vi "Calibrate_Plates.vi"() -> ()   [LabVIEW 2013]
uses:
  <vilib>/rvi/interface/nirviOpenFPGA/nirviOpenFPGA.xnode
  <vilib>/rvi/interface/nirviReadWriteControl/nirviReadWriteControl.xnode
  NiFpgaLv.dll
  <vilib>/Utility/error.llb/Error Cluster From Error Code.vi
  <vilib>/rvi/interface/Simulation/niFpgaSimulationCallBeginRW.vi
  <vilib>/rvi/errors/niLvFpgaAdjustHostInterfaceError.vi
  <vilib>/rvi/interface/nirviMethod/nirviMethod.xnode
  <vilib>/FPGAPlugInAG/Dynamic/niLvFpga_Run_Dynamic.vi
  <vilib>/rvi/interface/nirviCloseFPGA/nirviCloseFPGA.xnode
  <vilib>/FPGAPlugInAG/Dynamic/niLvFpga_Close_Dynamic.vi
  FPGA Bitfiles/ProjetoTasca_FPGATarget_ProjetoTASCA_c15+uw0dO0I.lvbitx
  ProjetoTASCA.vi
  <vilib>/rvi/interface/nirviMethod/StockFPGA_InlinedMethodWaitForSingleIRQ.vi
  <vilib>/FPGAPlugInAG/Dynamic/niLvFpga_WaitOnIrq_Dynamic.vi
  <vilib>/FPGAPlugInAG/cRIO-9075/niLvFpga_Open_cRIO-9075.vi
  <vilib>/rvi/interface/common/dynamic/niFpgaDynamicAddResources.vi
panel:
  in  "Passo da placa":dbl=0.5 format="%#_13g"
  out "Posicao da Placa":dbl format="%#_13g"
  in  "Arquivo de Saida":path=path "C:/SteeringDistillation/Medidas"
  out "Contagens - Det. 1":u32
  in  "Measurement Time (s)":sgl=1.0
  in  "Placa a calibrar":u16=1
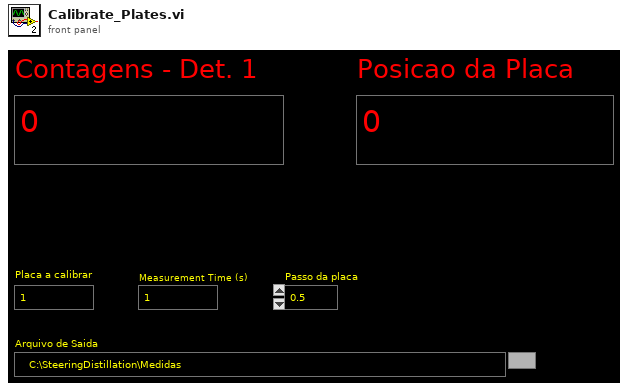
[diagram p1: front panel]
types:
  T1 = enum16{"open", "replace", "create", "open or create", "replace or create", "replace or create with confirmation"}
  T2 = cluster{"connection TCP":refnum<k5>, "LogTo File":bool, "Log File refnum":refnum<file>, "no error if error log":bool}
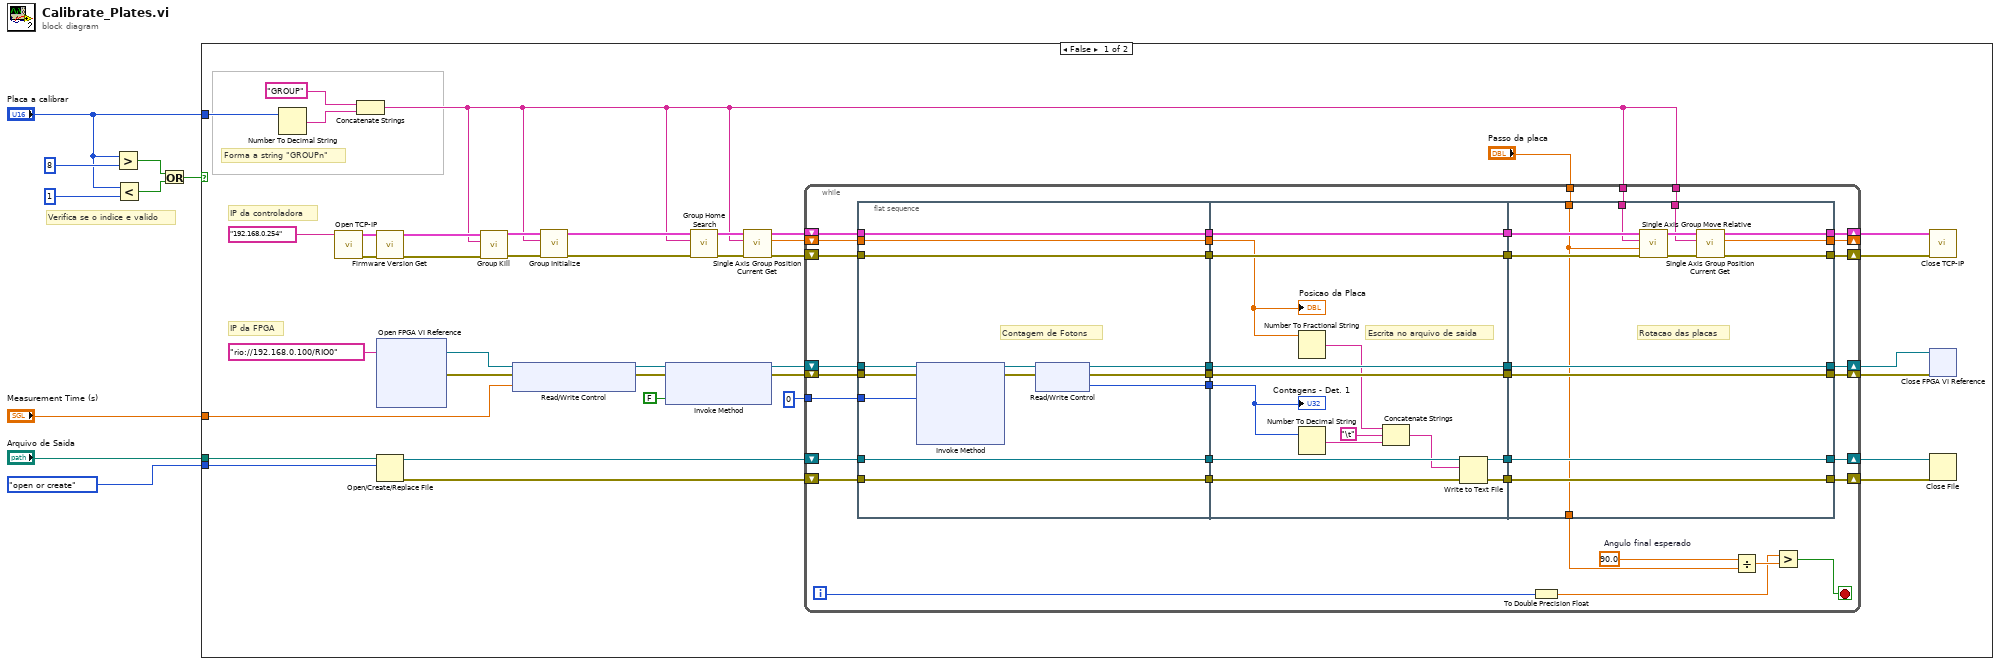
[diagram p0: block diagram]
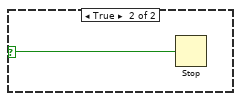
[diagram p2: hidden frame]
diagram:
  # "Verifica se o indice e valido"
  n1 = Greater?(x="Placa a calibrar", y=u16 8) -> (0:w7:bool)
  n2 = Less?(x="Placa a calibrar", y=u16 1) -> (x < y?=w6:bool)
  n3 = Or(x=w7, y=w6) -> (x .or. y?=w5:bool)
  n4 = case shown="False" w5 {
    selector: w5 -> [_ w126]
    tunnel: "Placa a calibrar" -> [w46 _]
    tunnel: "Measurement Time (s)" -> [w31 _]
    tunnel: T1."open or create" -> [w21 _]
    tunnel: "Arquivo de Saida" -> [w20 _]
    frame False {
      # "IP da FPGA"
      # "Forma a string \"GROUPn\""
      # "IP da controladora"
      n5 = Number To Decimal String(number=w46) -> (decimal integer string=w48:string)  [unwired: 1 in]
      n6 = call <userlib>:"Open TCP-IP.vi"("address"="192.168.0.254") -> ("error out"=w44:errorcluster, "Connection ID"=w43:T2)  [unwired: 8 in, 1 out]
      n7 = Concatenate Strings("GROUP" ("Group Name (250 c max)"), w48) -> (w10:string)
      n8 = call <userlib>:"Firmware Version Get.vi"("error in (no error)"=w44, "connection ID in"=w43) -> ("error out"=w41:errorcluster, "connection ID out"=w42:T2)  [unwired: 6 in, 2 out]
      n9 = xnode "Open FPGA VI Reference"("resource name"=tag "rio://192.168.0.100/RIO0") -> ("FPGA VI Reference Out"=w36:refnum<k20>, "error out"=w35:errorcluster)  [unwired: 1 in]
      n10 = Open/Create/Replace File(file path (use dialog)=w20, operation (0:open)=w21) -> (refnum out=w22:refnum<file>, error out=w23:errorcluster)  [unwired: 4 in, 1 out]
      n11 = call <userlib>:"Group Kill.vi"("error in (no error)"=w41, "Group Name (250 c max)"=w10, "connection ID in"=w42) -> ("error out"=w39:errorcluster, "connection ID out"=w40:T2)  [unwired: 6 in, 1 out]
      n12 = xnode "Read/Write Control"("FPGA VI Reference In"=w36, "error in"=w35, "Measurement Time (s)"=w31) -> ("FPGA VI Reference Out"=w34:refnum<k20>, "error out"=w33:errorcluster)
      n13 = call <userlib>:"Group Initialize.vi"("error in (no error)"=w39, "Group Name (250 c max)"=w10, "connection ID in"=w40) -> ("error out"=w11:errorcluster, "connection ID out"=w38:T2)  [unwired: 6 in, 1 out]
      n14 = xnode "Invoke Method"("FPGA VI Reference In"=w34, "error in"=w33, "Wait Until Done (F)"=FALSE) -> ("FPGA VI Reference Out"=w27:refnum<k20>, "error out"=w28:errorcluster)
      n15 = call <userlib>:"Group Home Search.vi"("error in (no error)"=w11, "Group Name (250 c max)"=w10, "connection ID in"=w38) -> ("error out"=w16:errorcluster, "connection ID out"=w17:T2)  [unwired: 6 in, 1 out]
      n16 = call <userlib>:"Single Axis Group Position Current Get.vi"("error in (no error)"=w16, "Group  Name (250 c max)"=w10, "connection ID in"=w17) -> ("error out"=w14:errorcluster, "Current Position (units)"=w13:dbl, "connection ID out"=w15:T2)  [unwired: 5 in, 1 out]
      n17 = while {
        tunnel: w10 -> [w81]
        tunnel: w10 -> [w76]
        tunnel: 0 ("IRQ Number(s)") -> [w86]
        shift-right: [w85] -> w29
        shift-left: w28 -> [w84]
        shift-right: [w82] -> w26
        shift-left: w27 -> [w83]
        shift-right: [w78] -> w25
        shift-left: w22 -> [w80]
        shift-right: [w77] -> w24
        shift-left: w23 -> [w79]
        shift-right: [w73] -> w19
        shift-left: w15 -> [w74]
        shift-right: [w72] -> w18
        shift-left: w14 -> [w75]
        shift-right: [w57] -> _
        shift-left: w13 -> [w71]
        tunnel: "Passo da placa" -> [w56]
        i -> [w50]
        stop <- w51 stop-if-true
        w54 = 90.0  # Angulo final esperado
        n18 = flat-sequence {
          tunnel: w83 -> [w97]
          tunnel: w84 -> [w96]
          tunnel: w80 -> [w89]
          tunnel: w79 -> [w88]
          tunnel: w86 -> [w95]
          tunnel: [w89] -> w70
          tunnel: [w88] -> w68
          tunnel: [w94] -> w66
          tunnel: [w93] -> w64
          tunnel: w74 -> [w92]
          tunnel: [w92] -> w62
          tunnel: [w91] -> w60
          tunnel: w75 -> [w91]
          tunnel: w71 -> [w90]
          tunnel: [w90] -> w58
          tunnel: [w87] -> w55
          tunnel: w70 -> [w111]
          tunnel: [w111] -> w69
          tunnel: w68 -> [w110]
          tunnel: [w110] -> w67
          tunnel: w66 -> [w109]
          tunnel: [w109] -> w65
          tunnel: w64 -> [w108]
          tunnel: [w108] -> w63
          tunnel: w62 -> [w107]
          tunnel: [w107] -> w61
          tunnel: w60 -> [w106]
          tunnel: [w106] -> w59
          tunnel: w58 -> [w103]
          tunnel: w55 -> [w102]
          tunnel: [w125] -> w78
          tunnel: w69 -> [w125]
          tunnel: [w124] -> w77
          tunnel: w67 -> [w124]
          tunnel: [w123] -> w82
          tunnel: w65 -> [w123]
          tunnel: [w122] -> w85
          tunnel: w63 -> [w122]
          tunnel: w61 -> [w121]
          tunnel: w59 -> [w120]
          tunnel: w81 -> [w119]
          tunnel: [w116] -> w73
          tunnel: [w115] -> w72
          tunnel: w76 -> [w114]
          tunnel: [w113] -> w57
          tunnel: w56 -> [w112]
          tunnel: [w112] -> w53
          frame #0 {
            # "Contagem de Fotons"
            n19 = xnode "Invoke Method"("FPGA VI Reference In"=w97, "error in"=w96, "IRQ Number(s)"=w95) -> ("FPGA VI Reference Out"=w98:refnum<k20>, "error out"=w99:errorcluster)  [unwired: 1 in, 2 out]
            n20 = xnode "Read/Write Control"("FPGA VI Reference In"=w98, "error in"=w99) -> ("FPGA VI Reference Out"=w94:refnum<k20>, "error out"=w93:errorcluster, "Count 1"=w87:u32)
          }
          frame #1 {
            # "Escrita no arquivo de saida"
            n21 = Number To Fractional String(number=w103) -> (F-format string=w104:string)  [unwired: 3 in]
            n22 = Number To Decimal String(number=w102) -> (decimal integer string=w101:string)  [unwired: 1 in]
            n23 = Concatenate Strings(w104, "\t", w101) -> (w100:string)
            n24 = Write to Text File(text=w100) -> ()  [unwired: 3 in, 3 out]
            "Posicao da Placa" <- w103
            "Contagens - Det. 1" <- w102
          }
          frame #2 {
            # "Rotacao das placas"
            n25 = call <userlib>:"Single Axis Group Move Relative.vi"("error in (no error)"=w120, "Target Displacement (units)"=w112, "Group  Name (250 c max)"=w119, "connection ID in"=w121) -> ("error out"=w117:errorcluster, "connection ID out"=w118:T2)  [unwired: 6 in]
            n26 = call <userlib>:"Single Axis Group Position Current Get.vi"("error in (no error)"=w117, "Group  Name (250 c max)"=w114, "connection ID in"=w118) -> ("error out"=w115:errorcluster, "Current Position (units)"=w113:dbl, "connection ID out"=w116:T2)  [unwired: 5 in, 1 out]
          }
        }
        n27 = To Double Precision Float(number=w50) -> (double precision float=w49:dbl)
        n28 = Divide(x=w54, y=w53) -> (x/y=w52:dbl)
        n29 = Greater?(x=w49, y=w52) -> (0:w51:bool)
      }
      n30 = call <userlib>:"Close TCP-IP.vi"("error in (no error)"=w18, "connection ID in"=w19) -> ()  [unwired: 9 in, 1 out]
      n31 = xnode "Close FPGA VI Reference"("FPGA VI Reference In"=w26, "error in"=w29) -> ()  [unwired: 1 out]
      n32 = Close File(refnum=w25, error in=w24) -> ()  [unwired: 2 out]
    }
    frame True {
      n33 = Stop(stop? (T)=w126) -> ()
    }
  }
